vi "CounterGenerator.vi"() -> ()   [LabVIEW 2013]
uses:
  Data.lvclass/Data.lvclass/Data.ctl
  Singleton.lvclass/Singleton.lvclass/Singleton.ctl
  Singleton.lvclass/WriteDataVariant.vi
  Singleton.lvclass/ReadDataVariant.vi
  Singleton.lvclass/InstanceDestroy.vi
  Singleton.lvclass/Constructor.vi
  Singleton.lvclass/Destructor.vi
  Data.lvclass/Data.lvclass
panel:
  in  "Timeout":i32=1000
  out "Counter":i32
  # "我是計數產生器"
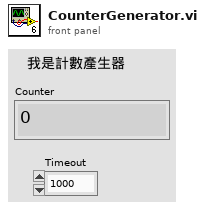
[diagram p1: front panel]
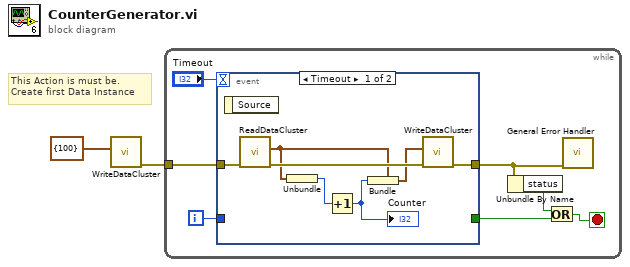
[diagram p0: block diagram]
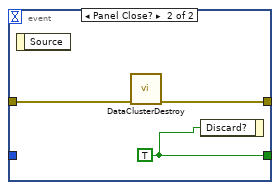
[diagram p2: hidden frame]
diagram:
  # "This Action is must be.\nCreate first Data Instance"
  n1 = call "WriteDataCluster.vi"("DataCluster"=cluster{"CounterNum":i32} {"CounterNum"=100}) -> ("error out"=w2:errorcluster)  [unwired: 10 in]
  n2 = while {
    tunnel: w2 -> [w3]
    i -> [w9]
    stop <- w4 stop-if-true
    n3 = event shown="[0] Timeout" {
      selector: _ -> [_ _]
      dyn-events: _ -> [_ _]
      timeout: "Timeout" -> [_ _]
      tunnel: w9 -> [_ _]
      tunnel: [_ w19] -> w5
      tunnel: [w12 w17] -> w6
      tunnel: w3 -> [w11 w18]
      event Timeout {
        n4 = event-data() -> ()  [unwired: 1 in, 1 out]
        n5 = call "ReadDataCluster.vi"("error in (no error)"=w11) -> ("error out"=w16:errorcluster, "DataCluster"=w15:cluster{"CounterNum":i32})  [unwired: 9 in]
        n6 = Unbundle(w15) -> ("CounterNum"=w13:i32)
        n7 = Increment(x=w13) -> (x+1=w10:i32)
        "Counter" <- w10
        n8 = Bundle(cluster=w15, "CounterNum"=w10) -> (w14:cluster{"CounterNum":i32})
        n9 = call "WriteDataCluster.vi"("error in (no error)"=w16, "DataCluster"=w14) -> ("error out"=w12:errorcluster)  [unwired: 9 in]
      }
      event Panel Close? {
        w19 = TRUE
        n10 = event-data() -> ()  [unwired: 1 in, 1 out]
        n11 = call "DataClusterDestroy.vi"("error in (no error)"=w18) -> ("error out"=w17:errorcluster)  [unwired: 10 in]
        n12 = event-data("Discard?"=w19) -> ()  [unwired: 1 in, 1 out]
      }
    }
    n13 = Unbundle By Name(w6) -> ("status"=w7:bool)
    n14 = Or(x=w7, y=w5) -> (x .or. y?=w4:bool)
    n15 = call <vilib>:"General Error Handler.vi"("error in (no error)"=w6) -> ()  [unwired: 10 in, 5 out]
  }
